vi "Write NI6008 Device Name.vi"(8 "error in (no error)":errorcluster, 10 "NI6008 Device Name":tag, 11 "Unit_Test_NI6008 in":refnum<class "Unit_Test_NI6008.lvclass">) -> (0 "error out":errorcluster, 3 "Unit_Test_NI6008 out":refnum<class "Unit_Test_NI6008.lvclass">)   [LabVIEW 2020, in "Unit_Test_NI6008.lvlib" / "Unit_Test_NI6008.lvclass"]
uses:
  Unit_Test_NI6008.lvclass
  Unit_Test_NI6008.lvclass/Unit_Test_NI6008.ctl
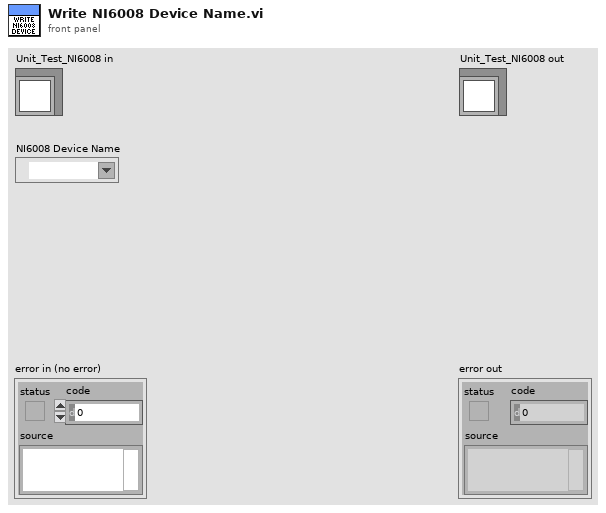
[diagram p1: front panel]
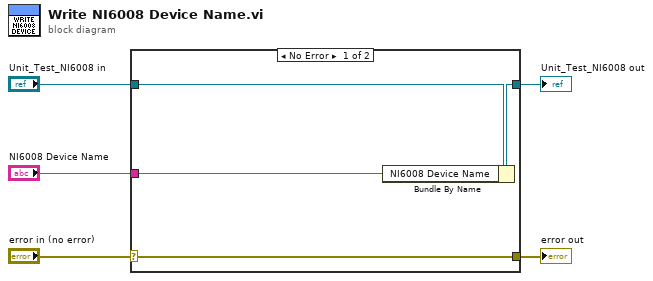
[diagram p0: block diagram]
diagram:
  n1 = case shown="No Error" "error in (no error)" {
    selector: "error in (no error)" -> [w9 w10]
    tunnel: [w9 w10] -> w4
    tunnel: [w7 w11] -> w2
    tunnel: "Unit_Test_NI6008 in" -> [w8 w11]
    tunnel: "NI6008 Device Name" -> [w6 _]
    frame No Error {
      n2 = Bundle By Name(cluster=w8, "NI6008 Device Name"=w6) -> (w7:refnum<class "Unit_Test_NI6008.lvclass">)
    }
    frame Error {
    }
  }
  "error out" <- w4
  "Unit_Test_NI6008 out" <- w2
